vi "Actor Core.vi"(8 "error in":cluster{"状态":bool, "代码":i32, "源":string} caption="错误输入", 11 "冷却器UI":refnum<class "Programmatic Controller.lvclass">) -> (0 "error out":cluster{"状态":bool, "代码":i32, "源":string} caption="错误输出", 3 "操作者输出":refnum<class "Actor.lvclass">)   [LabVIEW 2013, in "Programmatic Controller.lvclass"]
doc: "Actor Core.vi包含操作者的主要消息处理循环。操作者通常位于该循环中，在各种消息到达时对消息进行处理。如Do.vi消息返回任何错误，该循环将停止运行，错误代码43将被作为“无错误停止”的标准信号发送给调用方。如需更改上述行为，可在子孙类的Handle Error.vi中对该部分逻辑进行重写。"
uses:
  Programmatic Controller.lvclass
  <vilib>/ActorFramework/Actor/Actor.lvclass
  <vilib>/ActorFramework/Actor/Actor.lvclass/Actor.ctl
  <vilib>/ActorFramework/Message Enqueuer/Message Enqueuer.lvclass/Message Enqueuer.ctl
  Air Cooler Application/Load Into Sub Panel Msg/Load Into Sub Panel Msg.lvclass/Load Into Sub Panel Msg.ctl
  Programmatic Controller.lvclass/Programmatic Controller.ctl
  Cooler Controller/Cooler Controller/Cooler Controller.lvclass
  Cooler Controller/Change Desired Temperature Msg/Change Desired Temperature Msg.lvclass/Change Desired Temperature Msg.ctl
  <vilib>/ActorFramework/Message Enqueuer/Init from Existing Queue.vi
  <vilib>/ActorFramework/Message Enqueuer/Enqueue.vi
  <vilib>/ActorFramework/Message Priority Queue/Priority Enqueue.vi
  <vilib>/ActorFramework/Message Enqueuer/Message Enqueuer.lvclass
  Air Cooler Application/Load Into Sub Panel Msg/Load Into Sub Panel Msg.lvclass
  <vilib>/ActorFramework/Stop Msg/Stop Msg.lvclass
  Cooler Controller/Change Desired Temperature Msg/Change Desired Temperature Msg.lvclass
panel:
  in  "时间显示":string="%1.2f秒"
  out "已用时间":string
  out "编程设定的序列":enum32{"步骤1", "步骤2", "步骤3", "步骤4"}(radio)
  out "事件记录":string
  in  "停止":bool
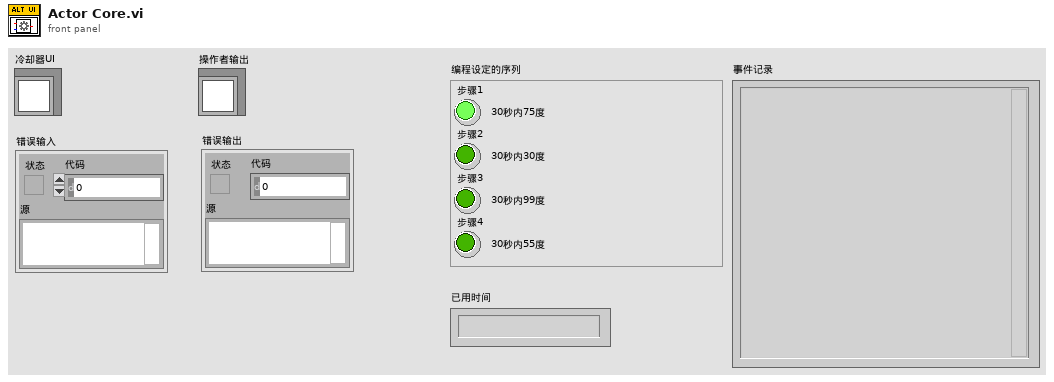
[diagram p1: front panel]
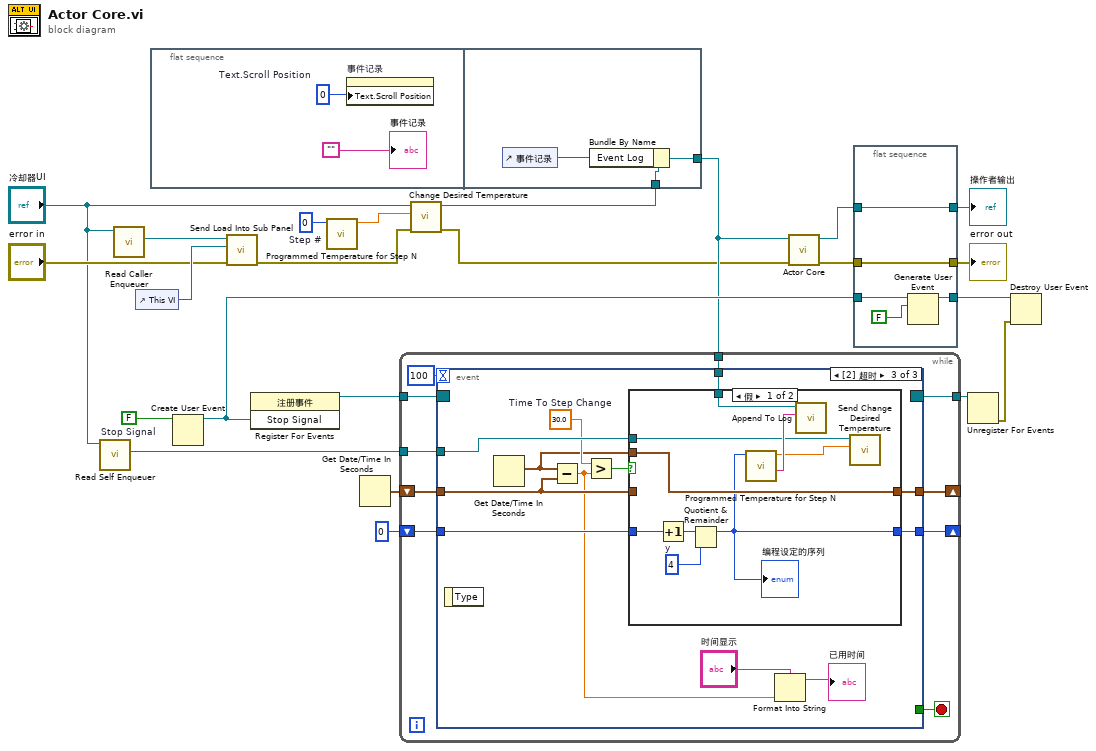
[diagram p0: block diagram]
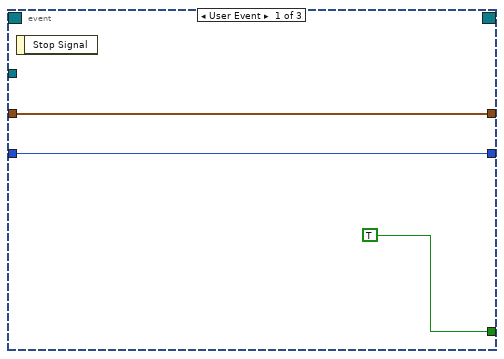
[diagram p2: hidden frame]
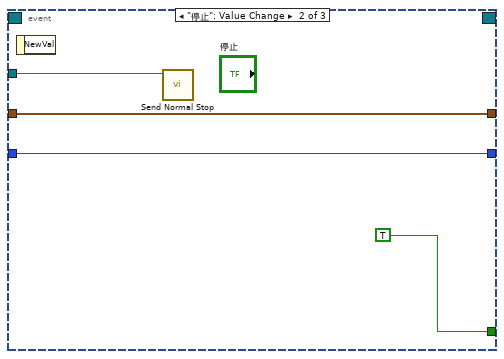
[diagram p3: hidden frame]
diagram:
  w8 = 0  # Step #
  w15 = FALSE  # Stop Signal
  n1 = call <vilib>:"Read Self Enqueuer.vi"("Actor"="冷却器UI") -> ("Self Enqueuer"=w6:refnum<class "Message Enqueuer.lvclass">)  [unwired: 10 in]
  n2 = call <vilib>:"Read Caller Enqueuer.vi"("Actor"="冷却器UI") -> ("Caller Enqueuer"=w13:refnum<class "Message Enqueuer.lvclass">)  [unwired: 10 in]
  n3 = control-ref of="This VI"() -> (w12:refnum<vi>)
  n4 = flat-sequence {
    tunnel: w4 -> [w28]
    tunnel: [w26] -> w7
    frame #0 {
      w25 = u32 0  # Text.Scroll Position
      n5 = property on="事件记录" class="Str"("Text.Scroll Position"=w25) -> ()  [unwired: 2 in, 2 out]
      "事件记录" <- ""
    }
    frame #1 {
      n6 = control-ref of="事件记录"() -> (w27:refnum<vi>)
      n7 = Bundle By Name(cluster=w28, "Event Log"=w27) -> (w26:refnum<class "Programmatic Controller.lvclass">)
    }
  }
  n8 = Create User Event(user event datatype=w15) -> (user event=w20:refnum<user-event>)  [unwired: 1 in, 1 out]
  n9 = call "Send Load Into Sub Panel.vi"("error in (no error)"="error in", "用于子面板的VI"=w12, "消息待入队列"=w13) -> ("error out"=w2:cluster{"状态":bool, "代码":i32, "源":string})  [unwired: 8 in]
  n10 = register-events(w20) -> (reference out=w23:refnum<event-registration>)  [unwired: 2 in, 1 out]
  n11 = call "Programmed Temperature for Step N.vi"("步骤编号"=w8) -> ("待维持的温度"=w3:dbl)  [unwired: 9 in, 1 out]
  n12 = Get Date/Time In Seconds() -> (seconds since 1Jan1904=w10:timestamp)
  n13 = while {
    tunnel: w23 -> [w38]
    tunnel: [w37] -> w22
    tunnel: w6 -> [w35]
    shift-right: [w34] -> _
    shift-left: w10 -> [w33]
    shift-right: [w31] -> _
    shift-left: 0 -> [w32]
    tunnel: w7 -> [w30]
    stop <- w36 stop-if-true
    n14 = event shown="[2] 超时" {
      selector: w38 -> [_ _ _]
      dyn-events: [_ _ _] -> w37
      timeout: 100 -> [_ _ _]
      tunnel: [TRUE TRUE _] -> w36
      tunnel: w35 -> [_ w45 w57]
      tunnel: [w39 w42 w53] -> w34
      tunnel: w33 -> [w39 w42 w54]
      tunnel: w32 -> [w40 w43 w51]
      tunnel: [w40 w43 w52] -> w31
      tunnel: w30 -> [_ _ w49]
      event User Event {
        n15 = event-data() -> ()  [unwired: 1 in, 1 out]
      }
      event "停止": Value Change {
        n16 = event-data() -> ()  [unwired: 1 in, 1 out]
        n17 = call <vilib>:"Send Normal Stop.vi"("Message Enqueuer"=w45) -> ()  [unwired: 10 in, 1 out]
      }
      event Timeout {
        w56 = 30.0  # Time To Step Change
        n18 = event-data() -> ()  [unwired: 1 in, 1 out]
        n19 = Get Date/Time In Seconds() -> (seconds since 1Jan1904=w50:timestamp)
        n20 = Subtract(x=w50, y=w54) -> (x-y=w46:dbl)
        n21 = Greater?(x=w56, y=w46) -> (0:w55:bool)
        n22 = case shown="假" w55 {
          tunnel: w57 -> [w59 _]
          tunnel: w54 -> [_ w68]
          tunnel: [w66 w68] -> w53
          tunnel: [w62 w67] -> w52
          tunnel: w51 -> [w65 w67]
          tunnel: w50 -> [w66 _]
          tunnel: w49 -> [w61 _]
          frame False {
            w63 = 4  # y
            n23 = Increment(x=w65) -> (x+1=w64:i32)
            n24 = Quotient & Remainder(x=w64, y=w63) -> (x-y*floor(x/y)=w62:i32)  [unwired: 1 out]
            "编程设定的序列" <- w62
            n25 = call "Programmed Temperature for Step N.vi"("步骤编号"=w62) -> ("新的温度消息"=w60:string, "待维持的温度"=w58:dbl)  [unwired: 9 in]
            n26 = call "Append To Log.vi"("字符串"=w60, "冷却器备用UI输入"=w61) -> ()  [unwired: 9 in, 1 out]
            n27 = call "Send Change Desired Temperature.vi"("待维持的温度"=w58, "消息待入队列"=w59) -> ()  [unwired: 9 in, 1 out]
          }
          frame True {
          }
        }
        n28 = Format Into String(format string="时间显示", w46) -> (resulting string=→"已用时间":string)  [unwired: 2 in, 1 out]
      }
    }
  }
  n29 = call "Change Desired Temperature.vi"("error in (no error)"=w2, "待维持的温度"=w3, "冷却器的控制器输入"="冷却器UI") -> ("error out"=w1:cluster{"状态":bool, "代码":i32, "源":string}, "冷却器的控制器输出"=w4:refnum<class "Programmatic Controller.lvclass">)  [unwired: 7 in]
  n30 = call-parent "Actor Core.vi"("error in"=w1, "Actor in"=w7) -> ("error out"=w16:errorcluster, "Actor out"=w18:refnum<class "Actor.lvclass">)  [unwired: 8 in]
  n31 = flat-sequence {
    tunnel: [w73] -> w21
    tunnel: w20 -> [w72]
    tunnel: w18 -> [w71]
    tunnel: [w71] -> w19
    tunnel: w16 -> [w70]
    tunnel: [w70] -> w17
    frame #0 {
      n32 = Generate User Event(user event=w72, event data cluster=FALSE) -> (user event out=w73:refnum<user-event>)  [unwired: 2 in, 1 out]
    }
  }
  n33 = Unregister For Events(event registration refnum=w22) -> (error out=w14:errorcluster)  [unwired: 1 in]
  n34 = Destroy User Event(user event=w21, error in=w14) -> ()  [unwired: 1 out]
  "error out" <- w17
  "操作者输出" <- w19
